vi "Fault Table.vi"(0 "GEA2 Reference In":refnum<k24>, 5 "GEA Inputs":T2 {"Destination" format="%.0x"; "Source" format="%.0x"}, 7 "Clear Table Buffer?":bool, 9 "Standalone?":bool, 11 "Error In":errorcluster) -> (2 "TI0_Fault_ID_Status":string, 3 "TI2_Fault_ID_Status":string, 4 "GEA2 Reference Out":refnum<k24>, 6 "TI4_Fault_ID_Status":string, 10 "ERD Data Out":T1[](array[typedef]) {"ERD Number" format="%.0x"}, 13 "TI1_Fault_ID_Status":string, 14 "TI3_Fault_ID_Status":string, 15 "Error Out":errorcluster)   [LabVIEW 2016, in "TLMB.lvlib"]
uses:
  Projects/TLMB.lvlib
  Q:/Common/DLLs/GEA3/GeaCommunication.dll
  Common/DLLs/GEA3/GeaCommunication.dll
  Common/LabVIEW GEA2 Toolkit/LabVIEW_GEA2_Toolkit.lvlibp/type defs/Source_Destination.ctl
  Common/LabVIEW GEA2 Toolkit/LabVIEW_GEA2_Toolkit.lvlibp/type defs/ERD Read Data Out.ctl
  Common/LabVIEW GEA2 Toolkit/LabVIEW_GEA2_Toolkit.lvlibp/type defs/ERD Read Data In.ctl
  Common/LabVIEW GEA2 Toolkit/LabVIEW_GEA2_Toolkit.lvlibp/type defs/Data Type.ctl
  Common/LabVIEW GEA2 Toolkit/LabVIEW_GEA2_Toolkit.lvlibp/type defs/ERD Write Data In.ctl
  type defs/Fault_Table_Information.ctl
  Common/LabVIEW GEA2 Toolkit/LabVIEW_GEA2_Toolkit.lvlibp
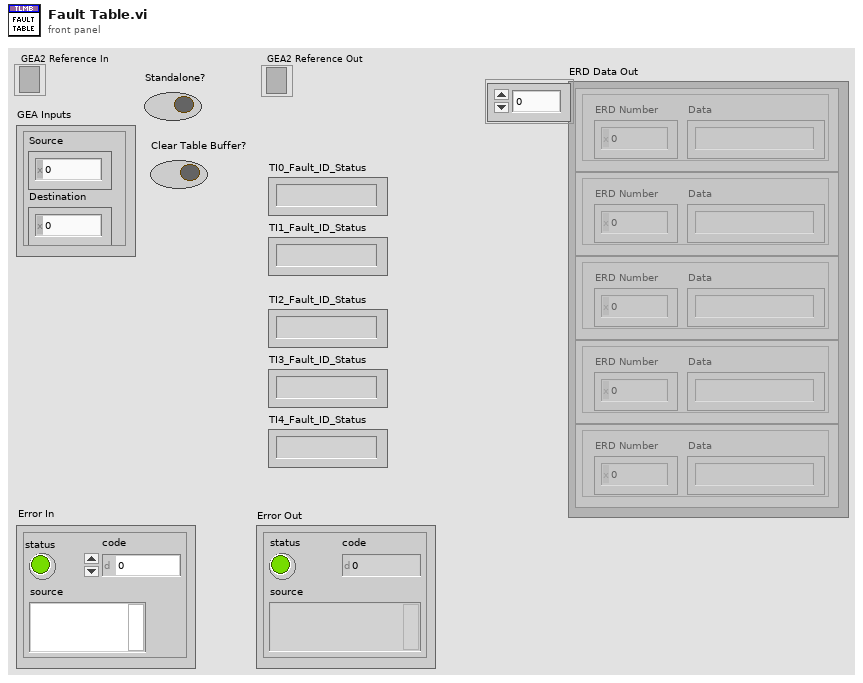
[diagram p1: front panel]
types:
  T1 = typedef "LabVIEW_GEA2_Toolkit.lvlibp/ERD Read Data Out.ctl" = cluster{"ERD Number":u16, "Data":string}
  T2 = typedef "LabVIEW_GEA2_Toolkit.lvlibp/Source_Destination.ctl" = cluster{"Source":u8, "Destination":u8}
  T3 = typedef "LabVIEW_GEA2_Toolkit.lvlibp/ERD Read Data In.ctl" = cluster{"ERD Number":u16, "Data Type":T4}
  T4 = typedef "LabVIEW_GEA2_Toolkit.lvlibp/Data Type.ctl" = enum16{"string", "boolean", "uint8_t", "uint16_t", "uint32_t", "uint64_t", "int8_t", "int16_t", "int32_t", "int64_t"}
  T5 = typedef "TLMB.lvlib/Fault_Table_Information.ctl" = cluster{"Cycle Count":u32, " Runtime (min) ":u32, "Fault ID":string, "Fault Count":u32, "Fault Status":string}
  T6 = typedef "LabVIEW_GEA2_Toolkit.lvlibp/ERD Write Data In.ctl" = cluster{"ERD Number":u16, "Data Type":T4, "Data":string}
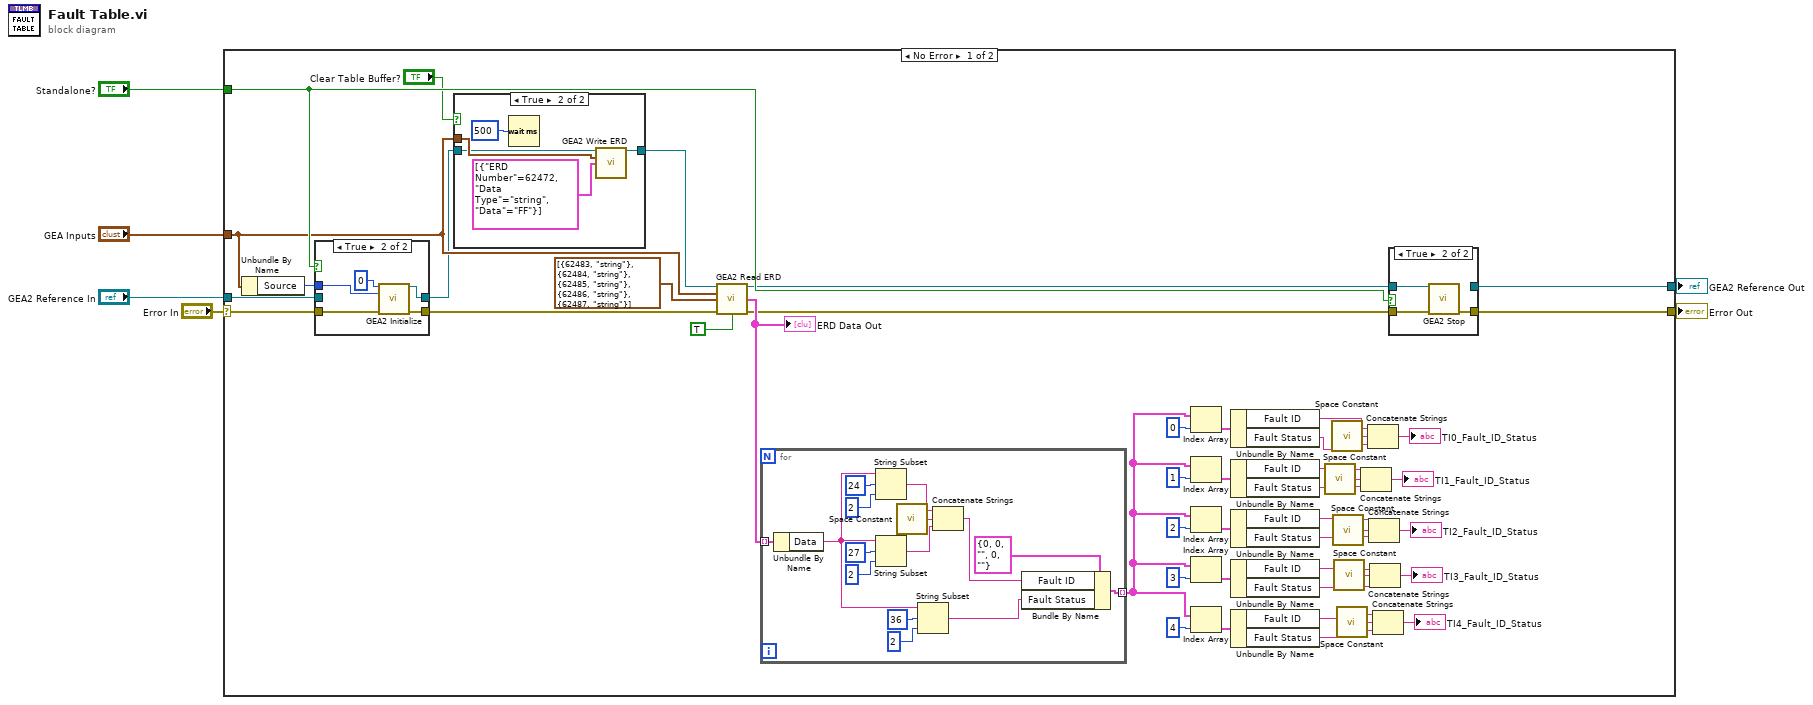
[diagram p0: block diagram]
diagram:
  n1 = case shown="No Error" "Error In" {
    selector: "Error In" -> [w53 w88]
    tunnel: [w50 w88] -> w6
    tunnel: [w51 w87] -> w5
    tunnel: "GEA Inputs" -> [w44 _]
    tunnel: "Standalone?" -> [w48 _]
    tunnel: "GEA2 Reference In" -> [w43 w87]
    frame No Error {
      n2 = Unbundle By Name(w44) -> ("Source"=w52:u8)
      n3 = case shown="True" w48 {
        tunnel: w53 -> [w81 w86]
        tunnel: [w81 w85] -> w49
        tunnel: [w80 w84] -> w42
        tunnel: w52 -> [_ w83]
        tunnel: w43 -> [w80 _]
        frame False {
        }
        frame True {
          n4 = call "GEA2 Initialize.vi"("Board Index"=0, "Source Address"=w83, "error in"=w86) -> ("GEA2 Reference Out"=w84:refnum<k24>, "error out"=w85:errorcluster)  [unwired: 10 in, 1 out]
        }
      }
      n5 = case shown="True" "Clear Table Buffer?" {
        tunnel: w44 -> [_ w73]
        tunnel: w42 -> [w69 w72]
        tunnel: [w69 w71] -> w41
        frame False {
        }
        frame True {
          n6 = Wait (ms)(milliseconds to wait=u32 500) -> ()  [unwired: 1 out]
          n7 = call "GEA2 Write ERD.vi"("GEA2 Reference In"=w72, "GEA Inputs"=w73, "Write ERD List"=T6[] [{"ERD Number"=62472, "Data Type"=enum."string", "Data"="FF"}]) -> ("GEA2 Reference Out"=w71:refnum<k24>)  [unwired: 10 in, 2 out]
        }
      }
      n8 = call "GEA2 Read ERD.vi"("GEA2 Reference In"=w41, "GEA Inputs"=w44, "Read ERD List"=T3[] [{"ERD Number"=62483, "Data Type"=enum."string"}, {"ERD Number"=62484, "Data Type"=enum."string"}, {"ERD Number"=62485, "Data Type"=enum."string"}, {"ERD Number"=62486, "Data Type"=enum."string"}, {"ERD Number"=62487, "Data Type"=enum."string"}], "Error In"=w49, "Verify ERD Response?"=TRUE) -> ("GEA2 Reference Out"=w33:refnum<k24>, "ERD Data Out"=w32:T1[], "Error Out"=w26:errorcluster)  [unwired: 7 in, 1 out]
      "ERD Data Out" <- w32
      n9 = for {
        tunnel: [w59] -> w34 mode=indexing
        tunnel: w32 -> [w56] mode=indexing
        n10 = Unbundle By Name(w56) -> ("Data"=w60:string)
        n11 = String Subset(string=w60, offset (0)=24, length (rest)=2 ("length (rest)")) -> (substring=w66:string)
        n12 = String Subset(string=w60, offset (0)=27, length (rest)=2 ("length (rest)")) -> (substring=w54:string)
        n13 = call <vilib>:"Space Constant.vi"() -> ("String"=w55:string)
        n14 = String Subset(string=w60, offset (0)=36, length (rest)=2 ("length (rest)")) -> (substring=w57:string)
        n15 = Concatenate Strings(w66, w55, w54) -> (w58:string)
        n16 = Bundle By Name(cluster=T5 {"Cycle Count"=0, " Runtime (min) "=0, "Fault ID"="", "Fault Count"=0, "Fault Status"=""} ("Fault Entry 2"), "Fault ID"=w58, "Fault Status"=w57) -> (w59:T5)
      }
      n17 = Index Array(array=w34, index=0) -> (element=w40:T5)
      n18 = Index Array(array=w34, index=1) -> (element=w31:T5)
      n19 = Index Array(array=w34, index=2) -> (element=w30:T5)
      n20 = Index Array(array=w34, index=3) -> (element=w29:T5)
      n21 = Index Array(array=w34, index=4) -> (element=w28:T5)
      n22 = Unbundle By Name(w40) -> ("Fault ID"=w27:string, "Fault Status"=w24:string)
      n23 = Unbundle By Name(w31) -> ("Fault ID"=w19:string, "Fault Status"=w18:string)
      n24 = Unbundle By Name(w30) -> ("Fault ID"=w17:string, "Fault Status"=w16:string)
      n25 = Unbundle By Name(w29) -> ("Fault ID"=w15:string, "Fault Status"=w14:string)
      n26 = Unbundle By Name(w28) -> ("Fault ID"=w13:string, "Fault Status"=w12:string)
      n27 = call <vilib>:"Space Constant.vi"() -> ("String"=w23:string)
      n28 = call <vilib>:"Space Constant.vi"() -> ("String"=w25:string)
      n29 = call <vilib>:"Space Constant.vi"() -> ("String"=w22:string)
      n30 = call <vilib>:"Space Constant.vi"() -> ("String"=w21:string)
      n31 = call <vilib>:"Space Constant.vi"() -> ("String"=w20:string)
      n32 = Concatenate Strings(w19, w23, w18) -> (→"TI1_Fault_ID_Status":string)
      n33 = Concatenate Strings(w27, w25, w24) -> (→"TI0_Fault_ID_Status":string)
      n34 = Concatenate Strings(w17, w22, w16) -> (→"TI2_Fault_ID_Status":string)
      n35 = Concatenate Strings(w15, w21, w14) -> (→"TI3_Fault_ID_Status":string)
      n36 = Concatenate Strings(w13, w20, w12) -> (→"TI4_Fault_ID_Status":string)
      n37 = case shown="True" w48 {
        tunnel: [w75 w78] -> w50
        tunnel: [w76 _] -> w51
        tunnel: w33 -> [w76 w79]
        tunnel: w26 -> [w75 w77]
        frame False {
        }
        frame True {
          n38 = call "GEA2 Stop.vi"("GEA2 Reference In"=w79, "Error In"=w77) -> ("Error Out"=w78:errorcluster)  [unwired: 13 in]
        }
      }
    }
    frame Error {
    }
  }
  "Error Out" <- w6
  "GEA2 Reference Out" <- w5
